vi "Read Pot.vi"(8 "error in (no error)":errorcluster, 11 "Potentiometer I2C In":refnum<class "Potentiometer I2C.lvclass">) -> (0 "error out":errorcluster, 2 "Pot Value(0-127)":u8, 3 "Potentiometer I2C out":refnum<class "Potentiometer I2C.lvclass">)   [LabVIEW 2020, in "CTI-Peripheral.lvlib" / "Potentiometer I2C.lvclass"]
uses:
  Potentiometer I2C.lvclass
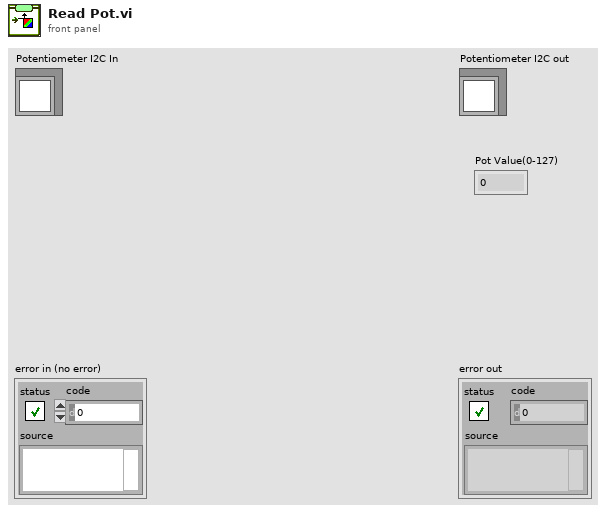
[diagram p1: front panel]
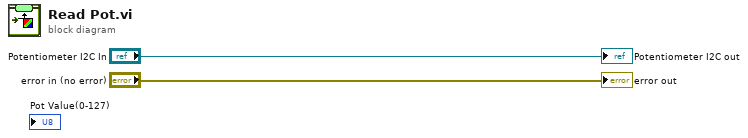
[diagram p0: block diagram]
diagram:
  "error out" <- "error in (no error)"
  "Potentiometer I2C out" <- "Potentiometer I2C In"
